vi "chart axis minor gridlines set visible.vi"(8 "error in (no error)":errorcluster, 10 "visible":u8, 11 "axis":u32) -> (0 "error out":errorcluster)   [LabVIEW 2015, in "xlsxwriter.lvlib"]
doc: "void chart_axis_minor_gridlines_set_visible(lxw_chart_axis axis, uint8_t visible);"
uses:
  xlsxwriter.lvlib
  xlsxwriter.dll
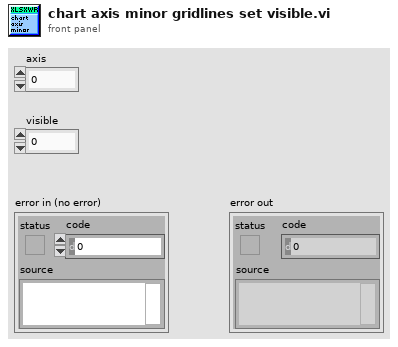
[diagram p1: front panel]
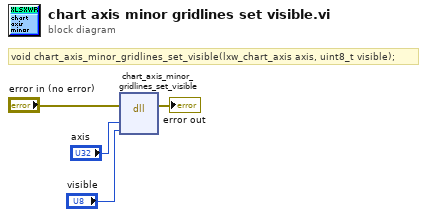
[diagram p0: block diagram]
diagram:
  # "void chart_axis_minor_gridlines_set_visible(lxw_chart_axis axis, uint8_t visible);"
  n1 = dll-call lib="C:/Users/WDAGUtilityAccount/Desktop/lv_vis_added_cell/xlsxwriter.*" fn="chart_axis_minor_gridlines_set_visible"(error in="error in (no error)", "axis"="axis", "visible"="visible") -> (error out=→"error out":errorcluster)  [unwired: 5 in, 1 out]
